vi "DataSocketServer-transmitter.vi"() -> ()   [LabVIEW 2020]
uses:
  <vilib>/numeric/Random Number (Range) I64.vi
  <vilib>/numeric/sub_Random U32.vi
panel:
  in  "stop":bool
  out "Waveform Chart":i64(graph)
  out "Numeric":i64
  out "Gauge":i64(knob) scale=0.0..100.0
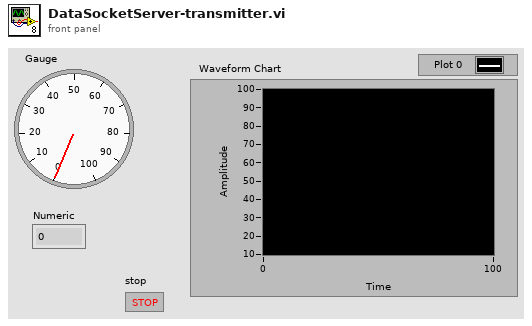
[diagram p1: front panel]
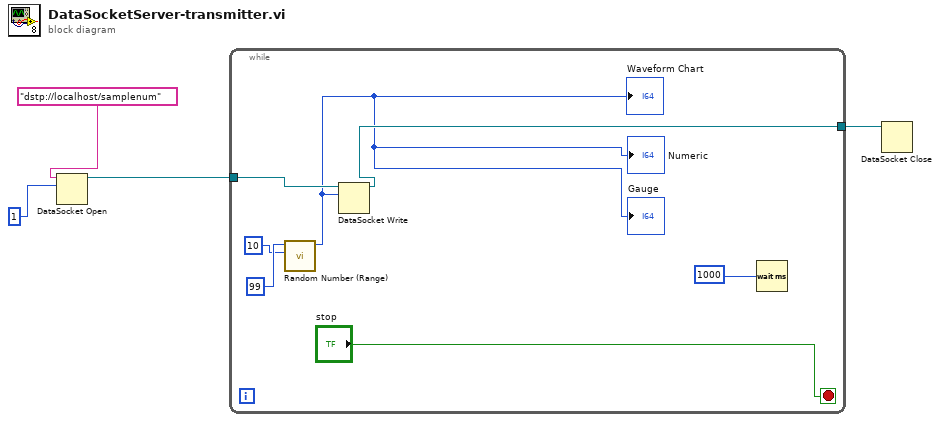
[diagram p0: block diagram]
diagram:
  n1 = DataSocket Open(10:1, 11:"dstp://localhost/samplenum") -> (3:w3:refnum<k13>)  [unwired: 2 in, 1 out]
  n2 = while {
    tunnel: w3 -> [w9]
    tunnel: [w8] -> w2
    stop <- "stop" stop-if-true
    n3 = call-poly <vilib>:"Random Number (Range).vi"("lower bound (-100)"=10, "upper bound (100)"=99) -> ("number"=w7:i64)  [unwired: 9 in]
    "Waveform Chart" <- w7
    "Numeric" <- w7
    "Gauge" <- w7
    n4 = DataSocket Write(10:w7, 11:w9) -> (3:w8:refnum<k13>)  [unwired: 2 in, 2 out]
    n5 = Wait (ms)(milliseconds to wait=1000) -> ()  [unwired: 1 out]
  }
  n6 = DataSocket Close(11:w2) -> ()  [unwired: 2 in, 2 out]
